vi "SaveStoppanniAvRAvC.vi"(5 "dtAccel":u8(ring)=3 items=["Accelerance", "Mobility", "Receptance", "Microphone", "Unknown"], 8 "nAverages":u32=12, 9 "fComplex":u32, 10 "file (use dialog)":path, 11 "Complex FRF":cluster{"t0":dbl, "dt":dbl, "Y":cdb[]}) -> (0 "AvR file":path)   [LabVIEW 2022 SP3]
panel:
  out "Header Info":T1
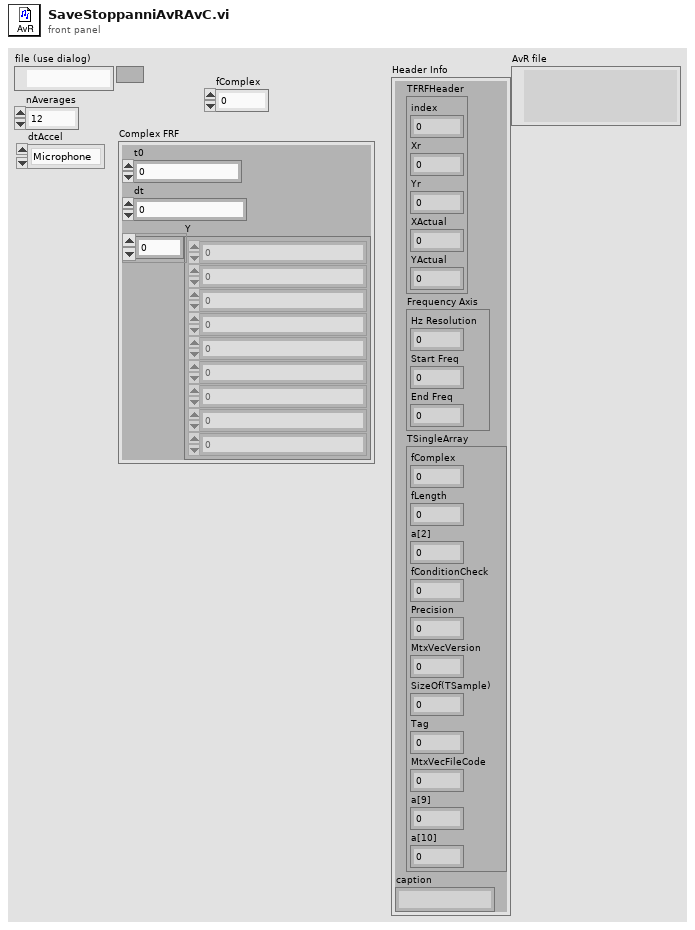
[diagram p1: front panel]
types:
  T1 = cluster{"TFRFHeader":cluster{"index":u32, "Xr":dbl, "Yr":dbl, "XActual":dbl, "YActual":dbl}, "Frequency Axis":cluster{"Hz Resolution":dbl, "Start Freq":dbl, "End Freq":dbl}, "TSingleArray":cluster{"fComplex":u32, "fLength":dbl, "a[2]":dbl, "fConditionCheck":dbl, "Precision":dbl, "MtxVecVersion":dbl, "SizeOf(TSample)":dbl, "Tag":dbl, "MtxVecFileCode":dbl, "a[9]":dbl, "a[10]":dbl}, "caption":string}
  T2 = enum16{"big-endian, network order", "native, host order", "little-endian"}
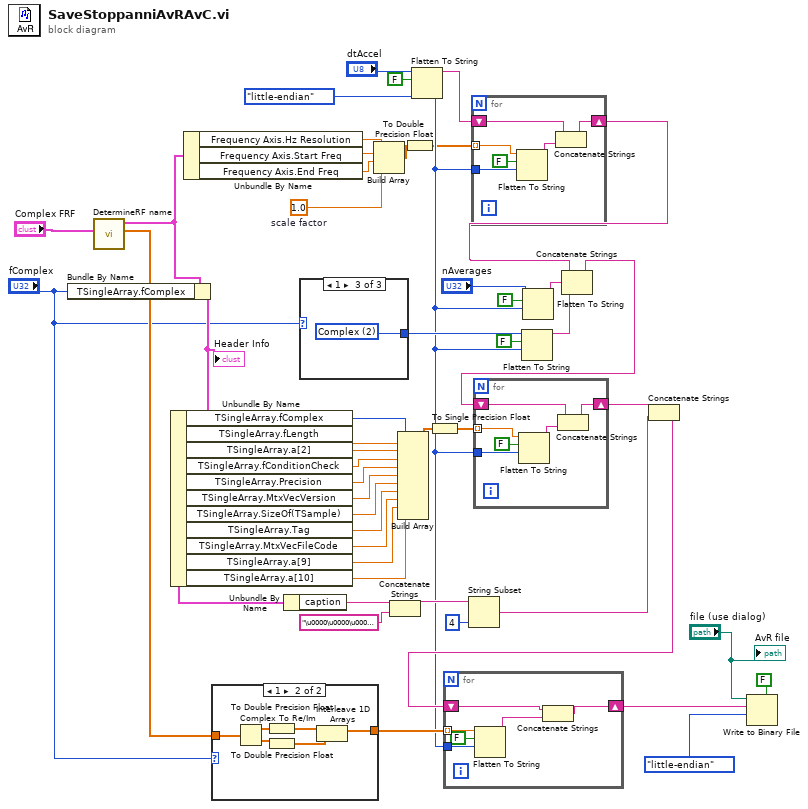
[diagram p0: block diagram]
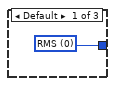
[diagram p2: hidden frame]
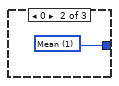
[diagram p3: hidden frame]
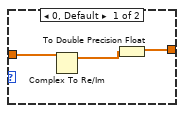
[diagram p4: hidden frame]
diagram:
  w16 = 1.0  # scale factor
  w4 = T2."little-endian" ("byte order (0:big-endian, network order)")
  n1 = call "DetermineRF name.vi"("Complex FRF"="Complex FRF") -> ("Y"=w18:cdb[], "Header Info"=w12:T1)  [unwired: 7 in, 2 out]
  n2 = Bundle By Name(cluster=w12, "TSingleArray.fComplex"="fComplex") -> (w11:T1)
  "Header Info" <- w11
  n3 = Unbundle By Name(w11) -> ("TSingleArray.fComplex"=w41:u32, "TSingleArray.fLength"=w40:dbl, "TSingleArray.a[2]"=w42:dbl, "TSingleArray.fConditionCheck"=w39:dbl, "TSingleArray.Precision"=w38:dbl, "TSingleArray.MtxVecVersion"=w37:dbl, "TSingleArray.SizeOf(TSample)"=w36:dbl, "TSingleArray.Tag"=w35:dbl, "TSingleArray.MtxVecFileCode"=w34:dbl, "TSingleArray.a[9]"=w33:dbl, "TSingleArray.a[10]"=w32:dbl)
  n4 = Unbundle By Name(w12) -> ("Frequency Axis.Hz Resolution"=w46:dbl, "Frequency Axis.Start Freq"=w47:dbl, "Frequency Axis.End Freq"=w45:dbl)
  n5 = case shown="1" "fComplex" {
    tunnel: [w49 w53] -> w27
    tunnel: w18 -> [w51 w52]
    frame 0, Default {
      n6 = Complex To Re/Im(x + iy=w51) -> (x=w50:dbl[])  [unwired: 1 out]
      n7 = To Double Precision Float(number=w50) -> (double precision float=w49:dbl[])
    }
    frame 1 {
      n8 = Complex To Re/Im(x + iy=w52) -> (x=w57:dbl[], y=w56:dbl[])
      n9 = To Double Precision Float(number=w57) -> (double precision float=w55:dbl[])
      n10 = To Double Precision Float(number=w56) -> (double precision float=w54:dbl[])
      n11 = Interleave 1D Arrays(w55, w54) -> (w53:dbl[])
    }
  }
  n12 = Unbundle By Name(w11) -> ("caption"=w29:string)
  n13 = case shown="1" "fComplex" {
    tunnel: [w58 w59 w60] -> w5
    frame Default {
      w58 = u8 0 items=["RMS", "Mean", "Complex", "Geometric", "None"] ("Average type")
    }
    frame 0 {
      w59 = u8 1 items=["RMS", "Mean", "Complex", "Geometric", "None"] ("Average type")
    }
    frame 1 {
      w60 = u8 2 items=["RMS", "Mean", "Complex", "Geometric", "None"] ("Average type")
    }
  }
  n14 = Build Array(w46, w47, w45, w16) -> (w44:dbl[])
  n15 = Concatenate Strings(w29, "\u0000\u0000\u0000\u0000" ("string")) -> (w28:string)
  n16 = Build Array(w41, w40, w42, w39, w38, w37, w36, w35, w34, w33, w32) -> (w43:dbl[])
  n17 = To Double Precision Float(number=w44) -> (double precision float=w2:dbl[])
  n18 = Flatten To String(anything="dtAccel", prepend array or string size? (T)=FALSE, byte order (0:big-endian, network order)=w4) -> (data string=w17:string)  [unwired: 1 in, 2 out]
  n19 = To Single Precision Float(number=w43) -> (single precision float=w24:sgl[])
  n20 = String Subset(string=w28, length (rest)=4 ("length (rest)")) -> (substring=w23:string)  [unwired: 1 in]
  n21 = for {
    tunnel: w4 -> [w65]
    tunnel: w2 -> [w64] mode=indexing
    shift-right: [w61] -> w14
    shift-left: w17 -> [w63]
    n22 = Flatten To String(anything=w64, prepend array or string size? (T)=FALSE, byte order (0:big-endian, network order)=w65) -> (data string=w62:string)  [unwired: 1 in, 2 out]
    n23 = Concatenate Strings(w63, w62) -> (w61:string)
  }
  n24 = Flatten To String(anything=w5, prepend array or string size? (T)=FALSE, byte order (0:big-endian, network order)=w4) -> (data string=w3:string)  [unwired: 1 in, 2 out]
  n25 = Flatten To String(anything="nAverages", prepend array or string size? (T)=FALSE, byte order (0:big-endian, network order)=w4) -> (data string=w8:string)  [unwired: 1 in, 2 out]
  n26 = Concatenate Strings(w14, w8, w3) -> (w13:string)
  n27 = for {
    tunnel: w4 -> [w71]
    tunnel: w24 -> [w70] mode=indexing
    shift-right: [w67] -> w31
    shift-left: w13 -> [w69]
    n28 = Flatten To String(anything=w70, prepend array or string size? (T)=FALSE, byte order (0:big-endian, network order)=w71) -> (data string=w68:string)  [unwired: 1 in, 2 out]
    n29 = Concatenate Strings(w69, w68) -> (w67:string)
  }
  n30 = Concatenate Strings(w31, w23) -> (w26:string)
  n31 = for {
    tunnel: w27 -> [w77] mode=indexing
    tunnel: w4 -> [w73]
    shift-right: [w74] -> w20
    shift-left: w26 -> [w76]
    n32 = Flatten To String(anything=w77, prepend array or string size? (T)=FALSE, byte order (0:big-endian, network order)=w73) -> (data string=w75:string)  [unwired: 1 in, 2 out]
    n33 = Concatenate Strings(w76, w75) -> (w74:string)
  }
  n34 = Write to Binary File(file (use dialog)="file (use dialog)", data=w20, 5:FALSE ("prepend array or string size? (T)"), 9:T2."little-endian" ("byte order (0:big-endian, network order)")) -> ()  [unwired: 2 in, 3 out]
  "AvR file" <- "file (use dialog)"
